vi "wifiString.vi"(11 "wifiString":string) -> (3 "Closures":bool[](array[boolean]))   [LabVIEW 2015]
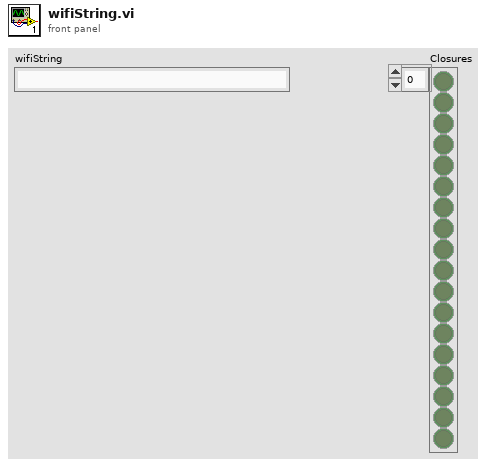
[diagram p1: front panel]
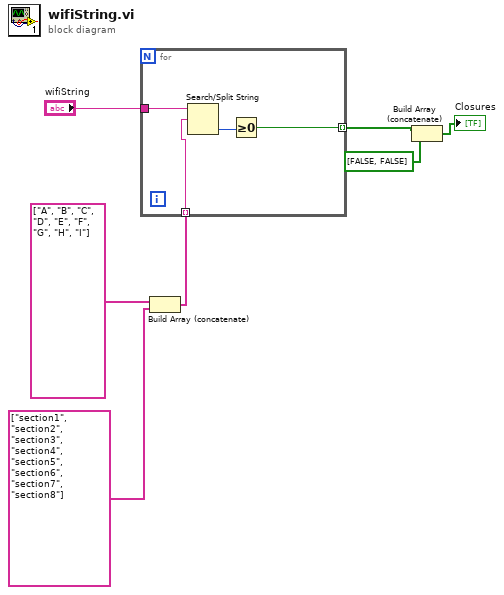
[diagram p0: block diagram]
diagram:
  n1 = Build Array (concatenate)(string[] ["A", "B", "C", "D", "E", "F", "G", "H", "I"], string[] ["section1", "section2", "section3", "section4", "section5", "section6", "section7", "section8"]) -> (w5:string[])
  n2 = for {
    tunnel: w5 -> [w10] mode=indexing
    tunnel: "wifiString" -> [w11]
    tunnel: [w8] -> w3 mode=indexing
    n3 = Search/Split String(string=w11, search string/char (-)=w10) -> (offset of match=w9:i32)  [unwired: 1 in, 2 out]
    n4 = Greater Or Equal To 0?(x=w9) -> (x >= 0?=w8:bool)
  }
  n5 = Build Array (concatenate)(w3, bool[] [FALSE, FALSE] ("array")) -> (→"Closures":bool[])
